vi "HTTP GET JSON.vi"(8 "error in (no error)":errorcluster, 11 "Generated URL":string) -> (0 "error out":errorcluster, 2 "headers":string, 3 "body":string)   [LabVIEW 2014, in "FIRST Events API.lvlib"]
uses:
  FIRST Events API.lvlib
  <vilib>/httpClient/LabVIEWHTTPClient.lvlib
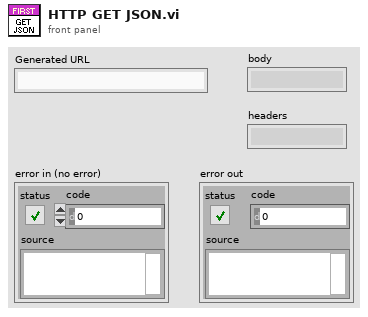
[diagram p1: front panel]
types:
  T1 = typedef "LabVIEWHTTPClient.lvlib/ClientHandle.ctl" = refnum<k1>
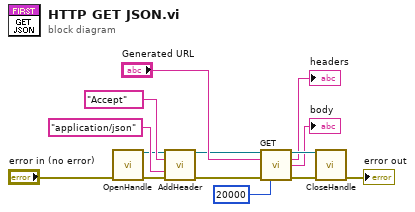
[diagram p0: block diagram]
diagram:
  n1 = call <vilib>:"OpenHandle.vi"("error in (no error)"="error in (no error)") -> ("client handle out"=w1:T1, "error out"=w2:errorcluster)  [unwired: 13 in]
  n2 = call <vilib>:"AddHeader.vi"("client handle"=w1, "header"="Accept", "value"="application/json", "error in (no error)"=w2) -> ("client handle out"=w5:T1, "error out"=w4:errorcluster)  [unwired: 10 in]
  n3 = call <vilib>:"GET.vi"("client handle"=w5, "url"="Generated URL", "error in (no error)"=w4, "timeout (10000)"=20000) -> ("client handle out"=w10:T1, "headers"=→"headers":string, "body"=→"body":string, "error out"=w11:errorcluster)  [unwired: 8 in]
  n4 = call <vilib>:"CloseHandle.vi"("client handle"=w10, "error in (no error)"=w11) -> ("error out"=→"error out":errorcluster)  [unwired: 13 in]
